vi "Print Error Message.vi"(8 "error in (no error)":errorcluster) -> ()   [LabVIEW 2020, in "Waveform Analog Output Engine.lvlib"]
uses:
  Waveform Analog Output Engine.lvlib
  <vilib>/Utility/error.llb/DialogType.ctl
  <vilib>/NI VeriStand/Custom Device Tools/Custom Device Utility Library/Custom Device Utility Library.lvlib
panel:
  out "message":string=" INSTRUCTIONS:\r\rNormal Use:  When using subVIs that incorporate the error in/error out (or error I/O) structure, place this handler where you want to inform the user of an error, typically at the end of the I/O data path, as the last action of the program.  If the error in error? is ERROR, the handler creates a message describing the error and its source.  If the type of dialog = 1 (default), the message is displayed to the user, who can only acknowedge it.  If the type = 2, the user can acknowledge the message or abort execution; aborting a program with active I/O is not recommended.  If the type = 0, no message is displayed; this is used to process the error programmatically, and the error out cluster elements are wired to individual terminals for that reason.  \r\rOther Use:\n\r\nlocal testing.  To test the error code of a subVI or function that does not have the error I/O structure, you can wire its error code and a source string to the local error code and error source inputs.  If error in error? indicates no error and error code is not equal to 0, the local code and source are substituted for the error in values, and error? is set TRUE (ERROR)."
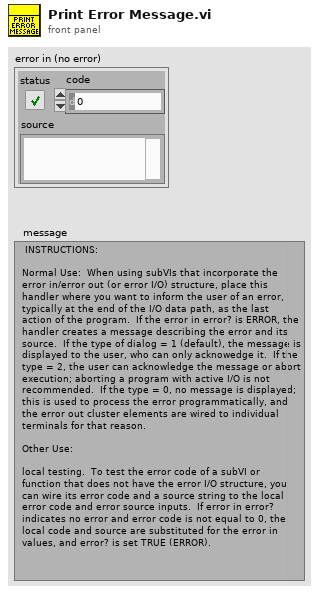
[diagram p1: front panel]
types:
  T1 = typedef "DialogType.ctl" = u16
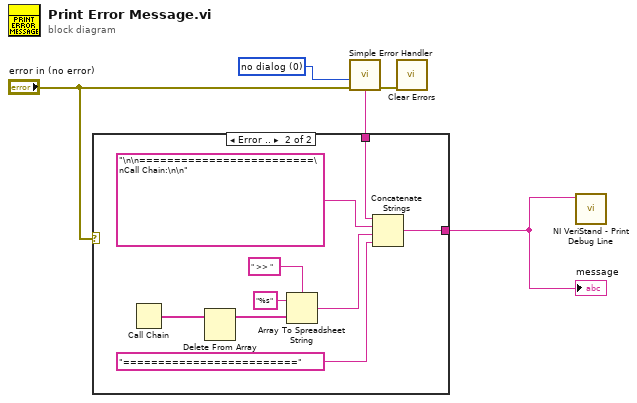
[diagram p0: block diagram]
diagram:
  w5 = T1 0 items=["no dialog", "OK message", "continue or stop message", "OK message + warnings", "continue/stop + warnings"] ("type of dialog (OK msg:1)")
  n1 = call <vilib>:"Simple Error Handler.vi"("type of dialog (OK msg:1)"=w5, "error in (no error)"="error in (no error)") -> ("error out"=w4:errorcluster, "message"=w3:string)  [unwired: 3 in, 3 out]
  n2 = case shown="Error .." "error in (no error)" {
    tunnel: w3 -> [w6 w12]
    tunnel: [w6 w9] -> w2
    frame No Error {
    }
    frame Error {
      n3 = Call Chain() -> (call chain=w15:string[])
      n4 = Delete From Array(array=w15) -> (array with subset deleted=w7:string[])  [unwired: 2 in, 1 out]
      n5 = Array To Spreadsheet String(delimiter (Tab)=" >> ", array=w7, 3:"%s" ("format string")) -> (spreadsheet string=w11:string)
      n6 = Concatenate Strings(w12, "\n\n=========================\nCall Chain:\n\n" ("string"), w11, "=========================" ("string")) -> (w9:string)
    }
  }
  "message" <- w2
  n7 = call <vilib>:"Clear Errors.vi"("error in (no error)"=w4) -> ()  [unwired: 5 in, 2 out]
  n8 = call <vilib>:"NI VeriStand - Print Debug Line.vi"("Message"=w2) -> ()  [unwired: 10 in, 1 out]
